vi "Initialize.vi"(8 "error in":errorcluster, 11 "Plugin in":refnum<class "Adjust Block Size.lvclass">) -> (0 "error out":errorcluster, 3 "Plugin out":refnum<class "Adjust Block Size.lvclass">)   [LabVIEW 2024, in "Adjust Block Size.lvlib" / "Adjust Block Size.lvclass"]
uses:
  Adjust Block Size.lvclass
  C:/Program Files/National Instruments/LabVIEW 2024/vi.lib/FlexLogger/SDK/PluginSDK.lvlibp/PEFClasses/SDK/Plugin/Plugin.lvclass
  <vilib>/FlexLogger/SDK/PluginSDK.lvlibp/PEFClasses/SDK/System Interface/Resampling Mode.ctl
  <vilib>/FlexLogger/SDK/PluginSDK.lvlibp/PEFClasses/SDK/Plugin/ParameterAccess/Write N Channel.vi
  <vilib>/FlexLogger/SDK/PluginSDK.lvlibp/PEFClasses/SDK/Plugin/ParameterAccess/Write DBL.vi
  <vilib>/FlexLogger/SDK/PluginSDK.lvlibp/PEFClasses/SDK/Plugin/Plugin.lvclass
  <vilib>/FlexLogger/SDK/PluginSDK.lvlibp/PEFClasses/SDK/System Interface/System Interface.lvclass
  C:/Program Files/National Instruments/LabVIEW 2024/vi.lib/FlexLogger/SDK/PluginSDK.lvlibp/PEFClasses/SDK/Processing Element/Processing Element.lvclass
  C:/dev/dsb/niflexlogger-plugins/PDK plugins/Adjust Block Size/Adjust Block Size.lvclass
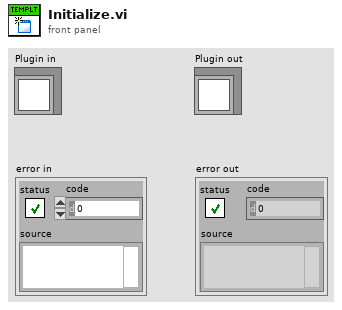
[diagram p1: front panel]
types:
  T1 = typedef "PluginSDK.lvlibp/System Interface.lvclass/Resampling Mode.ctl" = enum16{"No Resampling", "Custom Rate", "Maximum Rate", "Minimum Rate"}
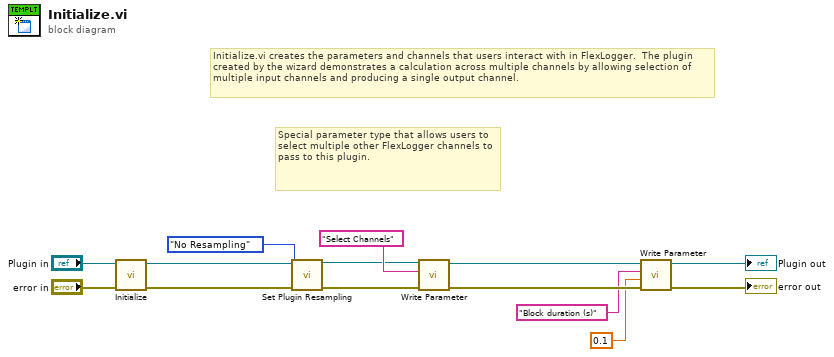
[diagram p0: block diagram]
diagram:
  # "Special parameter type that allows users to select multiple other FlexLogger channels to pass to this plugin."
  # "Initialize.vi creates the parameters and channels that users interact with in FlexLogger.  The plugin created by the wizard demonstrates a calculation across multiple channels by allowing selection of multiple input channels and producing a single output channel."
  n1 = call-parent "Initialize.vi"("error in (no error)"="error in", "Plugin in"="Plugin in") -> ("error out"=w10:errorcluster, "Plugin out"=w11:refnum<class "Adjust Block Size.lvclass">)  [unwired: 8 in]
  n2 = call <vilib>:"Set Plugin Resampling.vi"("Plugin in"=w11, "Resampling Mode"=Resampling_Mode."No Resampling", "error in (no error)"=w10) -> ("Plugin out"=w9:refnum<class "Adjust Block Size.lvclass">, "error out"=w8:errorcluster)  [unwired: 11 in]
  n3 = call-poly <vilib>:"Write Parameter.vi"("error in (no error)"=w8, "Name (Unique Channel Identifier)"="Select Channels" ("Name"), "Plugin in"=w9) -> ("error out"=w6:errorcluster, "Plugin out"=w7:refnum<class "Adjust Block Size.lvclass">)  [unwired: 7 in]
  n4 = call-poly <vilib>:"Write Parameter.vi"("error in (no error)"=w6, "Value"=0.1, "Name"="Block duration (s)", "Plugin in"=w7) -> ("error out"=→"error out":errorcluster, "Plugin out"=→"Plugin out":refnum<class "Adjust Block Size.lvclass">)  [unwired: 6 in]
